vi "ReadPicture.vi"(7 "PictureToRead":T9, 8 "error in":errorcluster, 10 "path to PNG file":path, 11 "InitCluster_IN":T1) -> (0 "error out":errorcluster, 3 "InitCluster_OUT":T1)   [LabVIEW 2022 SP3]
uses:
  SelectPictureToRead.ctl
  InitCluster.ctl
  CharacterCluster.ctl
  <vilib>/picture/picture.llb/imagedata.ctl
  ShotInitCluster.ctl
  <vilib>/Utility/miscctls.llb/LVPositionTypeDef.ctl
  <vilib>/Utility/miscctls.llb/LVBoundsTypeDef.ctl
  ShotCluster.ctl
  move_dir_ud.ctl
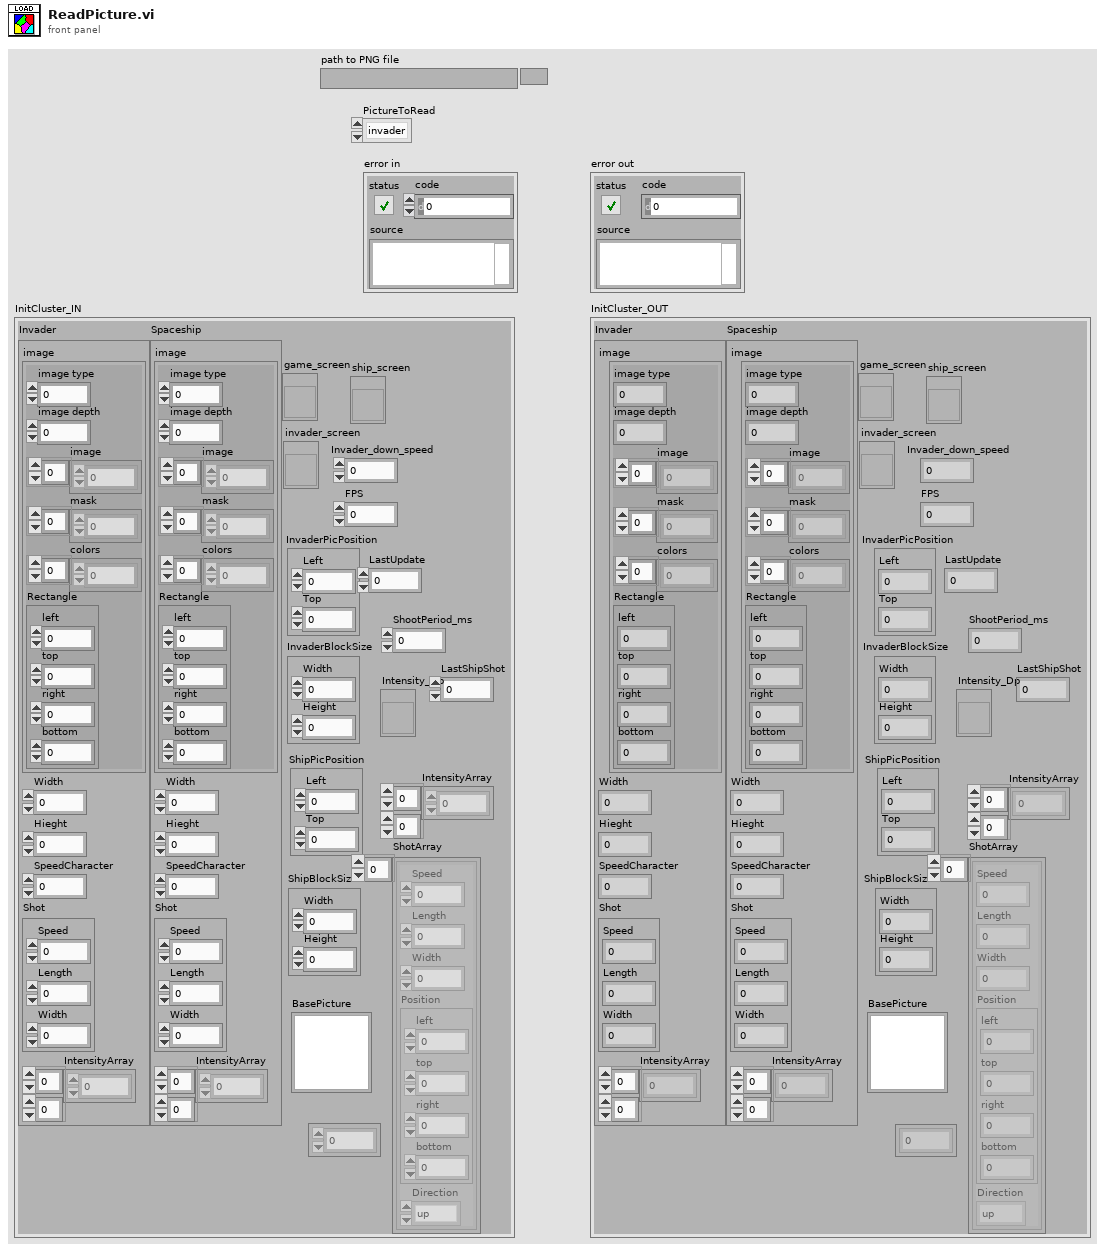
[diagram p1: front panel]
types:
  T1 = typedef "InitCluster.ctl" = cluster{"Invader":T2, "Spaceship":T2, "game_screen":refnum<vi>, "BasePicture":picture, "invader_screen":refnum<vi>, "InvaderPicPosition":T5, "Invader_down_speed":i16, "FPS":u16, "InvaderBlockSize":T6, "ship_screen":refnum<vi>, "ShipBlockSize":T6, "ShipPicPosition":T5, "LastUpdate":u32, "Intensity_Dp":refnum<vi>, "IntensityArray":u8[][], "ShotArray":T7[], "InvaderShotTimeArray":u32[], "ShootPeriod_ms":i32, "LastShipShot":u32}
  T2 = typedef "CharacterCluster.ctl" = cluster{"image":T3, "Width":u32, "Hieght":u32, "SpeedCharacter":u32, "Shot":T4, "IntensityArray":u8[][]}
  T3 = typedef "imagedata.ctl" = cluster{"image type":i32, "image depth":i32, "image":u8[], "mask":u8[], "colors":u32[], "Rectangle":cluster{"left":i16, "top":i16, "right":i16, "bottom":i16}}
  T4 = typedef "ShotInitCluster.ctl" = cluster{"Speed":u32, "Length":u32, "Width":u32}
  T5 = typedef "LVPositionTypeDef.ctl" = cluster{"Left":i32, "Top":i32}
  T6 = typedef "LVBoundsTypeDef.ctl" = cluster{"Width":u32, "Height":u32}
  T7 = typedef "ShotCluster.ctl" = cluster{"Speed":u32, "Length":u32, "Width":u32, "Position":cluster{"left":i16, "top":i16, "right":i16, "bottom":i16}, "Direction":T8}
  T8 = typedef "move_dir_ud.ctl" = enum16{"up", "down"}
  T9 = typedef "SelectPictureToRead.ctl" = enum16{"invader", "spaceship"}
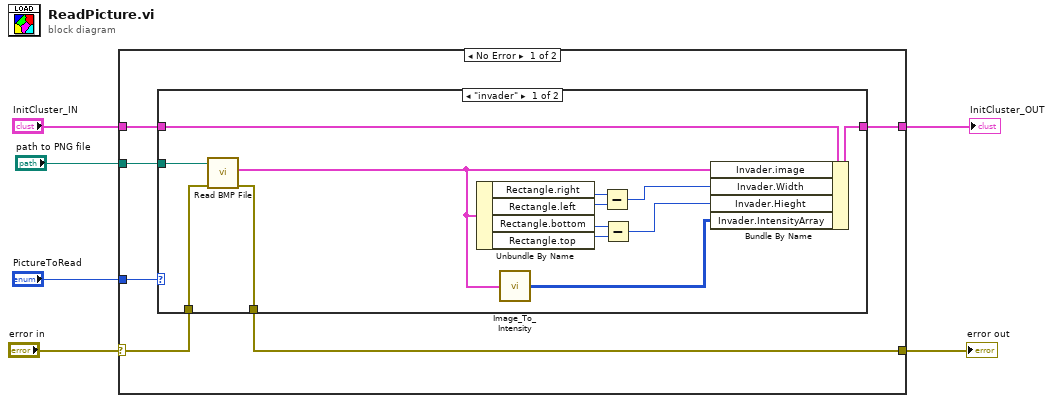
[diagram p0: block diagram]
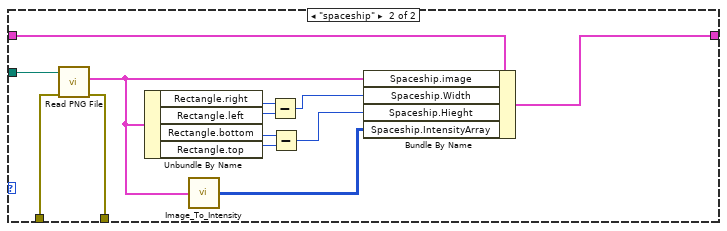
[diagram p2: hidden frame]
diagram:
  n1 = case shown="No Error" "error in" {
    selector: "error in" -> [w10 w39]
    tunnel: "PictureToRead" -> [w12 _]
    tunnel: "InitCluster_IN" -> [w11 w40]
    tunnel: [w9 w40] -> w3
    tunnel: [w8 w39] -> w2
    tunnel: "path to PNG file" -> [w7 _]
    frame No Error {
      n2 = case shown="\"invader\"" w12 {
        tunnel: w11 -> [w24 w37]
        tunnel: w10 -> [w25 w38]
        tunnel: [w23 w36] -> w9
        tunnel: [w22 w35] -> w8
        tunnel: w7 -> [w21 w34]
        frame "invader" {
          n3 = call <vilib>:"Read BMP File.vi"("error in (no error)"=w25, "path to BMP file"=w21) -> ("error out"=w22:errorcluster, "image data"=w14:T3)  [unwired: 7 in, 1 out]
          n4 = Unbundle By Name(w14) -> ("Rectangle.right"=w20:i16, "Rectangle.left"=w19:i16, "Rectangle.bottom"=w17:i16, "Rectangle.top"=w16:i16)
          n5 = call "Image_To_Intensity.vi"("image"=w14) -> ("Intensity Graph"=w13:u8[][])
          n6 = Subtract(x=w20, y=w19) -> (x-y=w18:i16)
          n7 = Subtract(x=w17, y=w16) -> (x-y=w15:i16)
          n8 = Bundle By Name(cluster=w24, "Invader.image"=w14, "Invader.Width"=w18, "Invader.Hieght"=w15, "Invader.IntensityArray"=w13) -> (w23:T1)
        }
        frame "spaceship" {
          n9 = call <vilib>:"Read PNG File.vi"("error in (no error)"=w38, "path to PNG file"=w34) -> ("error out"=w35:errorcluster, "image data"=w27:T3)  [unwired: 7 in, 1 out]
          n10 = Unbundle By Name(w27) -> ("Rectangle.right"=w33:i16, "Rectangle.left"=w32:i16, "Rectangle.bottom"=w30:i16, "Rectangle.top"=w29:i16)
          n11 = call "Image_To_Intensity.vi"("image"=w27) -> ("Intensity Graph"=w26:u8[][])
          n12 = Subtract(x=w33, y=w32) -> (x-y=w31:i16)
          n13 = Subtract(x=w30, y=w29) -> (x-y=w28:i16)
          n14 = Bundle By Name(cluster=w37, "Spaceship.image"=w27, "Spaceship.Width"=w31, "Spaceship.Hieght"=w28, "Spaceship.IntensityArray"=w26) -> (w36:T1)
        }
      }
    }
    frame Error {
    }
  }
  "error out" <- w2
  "InitCluster_OUT" <- w3
